vi "createSubFolder.vi"(8 "ErrorInput":errorcluster, 10 "FolderName":string) -> (0 "ErrorOutput":errorcluster)   [LabVIEW 2024]
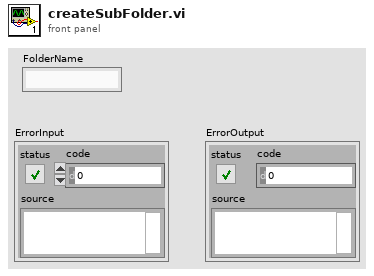
[diagram p1: front panel]
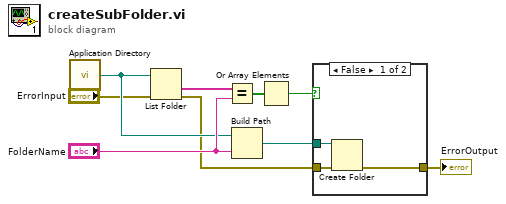
[diagram p0: block diagram]
diagram:
  n1 = call <vilib>:"Application Directory.vi"() -> ("Application Directory"=w6:path)
  n2 = List Folder(path=w6, error in="ErrorInput") -> (folder names=w3:string[], error out=w1:errorcluster)  [unwired: 2 in, 2 out]
  n3 = Equal?(x=w3, y="FolderName") -> (x = y?=w4:bool[])
  n4 = Build Path(base path=w6, name or relative path="FolderName") -> (appended path=w9:path)
  n5 = Or Array Elements(Boolean array=w4) -> (logical OR=w5:bool)
  n6 = case shown="False" w5 {
    tunnel: w9 -> [w12 _]
    tunnel: [w11 w13] -> w7
    tunnel: w1 -> [w10 w13]
    frame False {
      n7 = Create Folder(path (use dialog)=w12, error in=w10) -> (error out=w11:errorcluster)  [unwired: 1 in, 2 out]
    }
    frame True {
    }
  }
  "ErrorOutput" <- w7
